vi "Test View Stop Sent to View if Cleared while Running.vi"(8 "error in (no error)":errorcluster, 11 "View Test In":refnum<class "View Test.lvclass">) -> (0 "error out":errorcluster, 3 "View Test Out":refnum<class "View Test.lvclass">)   [LabVIEW 2020, in "View Test.lvclass"]
uses:
  View Test.lvclass
  C:/Program Files (x86)/National Instruments/LabVIEW 2020/vi.lib/Asteme/LUnit/Test Case.lvclass
  <vilib>/Asteme/LUnit/Test Case.lvclass/Test Case.ctl
  <vilib>/Asteme/LUnit/LUnit Assertion Result.lvclass/LUnit Assertion Result.ctl
  Support/Execution timer.vi
  <vilib>/Asteme/LUnit/Palette/Pass If.vi
  <vilib>/Asteme/LUnit/Set Assertion Type.vi
  <vilib>/Asteme/LUnit/Palette/Fail.vi
  <vilib>/Asteme/LUnit/Palette/Pass.vi
  <vilib>/Asteme/LUnit/LUnit Write Assertion Type.vi
  <vilib>/Asteme/LUnit/Add test result.vi
  <vilib>/Asteme/LUnit/LUnit Write Passed.vi
  <vilib>/Asteme/LUnit/LUnit Get Test Case.vi
  <vilib>/Asteme/LUnit/Assertion Result/LUnit Get Test Name.vi
  <vilib>/Asteme/LUnit/LUnit Write Message.vi
  <vilib>/Asteme/LUnit/LUnit Write Description.vi
  <vilib>/Asteme/LUnit/Read Test Case Name.vi
  Framework/View/View.lvclass
  C:/Users/anton/Documents/GitHub/Triarc-Framework/source/Framework/Process/Process.lvclass
  Support/Event Helpers/Dequeue Event Message.vi
  <vilib>/Asteme/LUnit/LUnit Assertion Result.lvclass
  Framework/Process/Process.lvclass
  Support/Event Helpers/Event Helpers.lvlib
  <vilib>/Asteme/LUnit/Test Case.lvclass
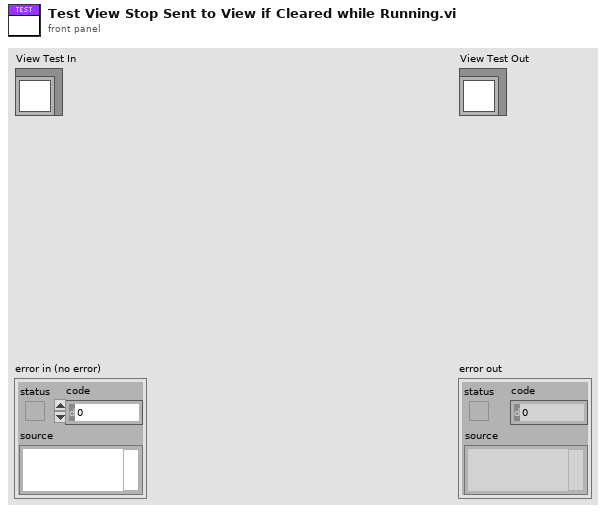
[diagram p1: front panel]
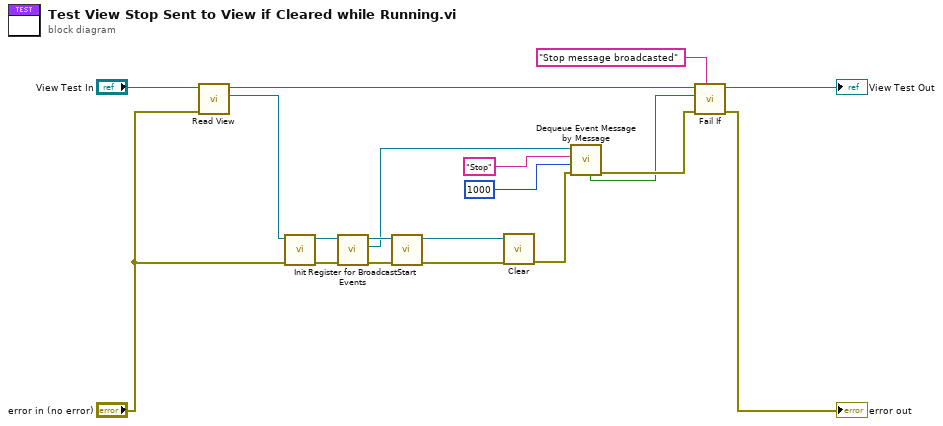
[diagram p0: block diagram]
diagram:
  n1 = call "Read View.vi"("error in (no error)"="error in (no error)", "View Test In"="View Test In") -> ("View"=w19:refnum<class "View.lvclass">, "View Test Out"=w4:refnum<class "View Test.lvclass">)  [unwired: 7 in, 1 out]
  n2 = call-dynamic "Init.vi"("error in (no error)"="error in (no error)", "View In"=w19) -> ("error out"=w16:errorcluster, "View Out"=w12:refnum<class "View.lvclass">)  [unwired: 8 in]
  n3 = call "Register for Broadcast Events.vi"("error in (no error)"=w16, "Process In"=w12) -> ("error out"=w13:errorcluster, "Event Registration Refnum Out"=w10:refnum<event-registration>, "Process Out"=w11:refnum<class "View.lvclass">)  [unwired: 7 in]
  n4 = call "Start.vi"("error in (no error)"=w13, "Process In"=w11) -> ("error out"=w14:errorcluster, "Process Out"=w15:refnum<class "View.lvclass">)  [unwired: 8 in]
  n5 = call-dynamic "Clear.vi"("error in (no error)"=w14, "View In"=w15) -> ("error out"=w9:errorcluster)  [unwired: 9 in]
  n6 = call "Dequeue Event Message by Message.vi"("error in (no error)"=w9, "Timeout (-1)"=1000, "Message"="Stop", "Event Registration Refnum"=w10) -> ("error out"=w8:errorcluster, "Timed Out?"=w2:bool)  [unwired: 3 in, 3 out]
  n7 = call <vilib>:"Fail If.vi"("Description"="Stop message broadcasted", "error in (no error)"=w8, "Fail?"=w2, "Test Case In"=w4) -> ("error out"=→"error out":errorcluster, "Test Case Out"=→"View Test Out":refnum<class "View Test.lvclass">)  [unwired: 6 in]
